vi "Draw Image Frame around marker.vi"(5 "Marker Index":i32, 7 "Camera Settings":T1, 9 "Altitude (m)":dbl, 11 "error in (no error)":errorcluster) -> (15 "error out":errorcluster)   [LabVIEW 2014]
uses:
  C:/Robotic Systems/Products/AgFalcon/Software/Ground Station/Data/Mapping DLL/GMap.NET.WindowsForms.dll
  Data/Mapping DLL/GMap.NET.WindowsForms.dll
  Lat Long Conversion/Controls/PointLatLon.ctl
  C:/Robotic Systems/Products/AgFalcon/Software/Ground Station/Data/Mapping DLL/GMap.NET.Core.dll
  Data/Mapping DLL/GMap.NET.Core.dll
  Reference/SubVI/Main Map Control Refernce.vi
  Settings File/Controls/Camera Settings.ctl
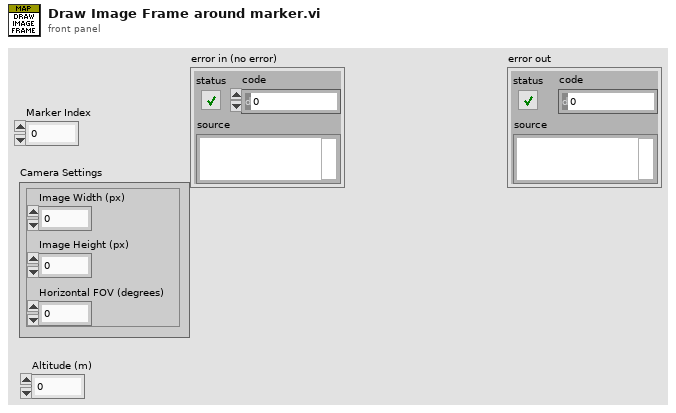
[diagram p1: front panel]
types:
  T1 = typedef "Camera Settings.ctl" = cluster{"Image Width (px)":dbl, "Image Height (px)":dbl, "Horizontal FOV (degrees)":dbl}
  T2 = typedef "PointLatLon.ctl" = cluster{"Longitude":dbl, "Latitude":dbl}
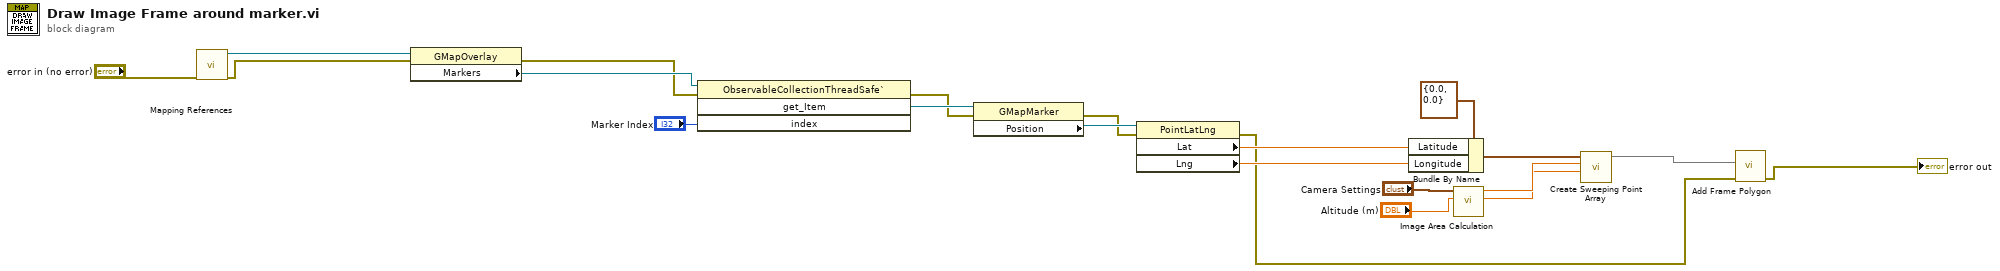
[diagram p0: block diagram]
diagram:
  n1 = call-poly "Mapping References.vi"("Error In"="error in (no error)") -> ("Error Out"=w3:errorcluster, "Main Map Reference"=w2:refnum<k24>)  [unwired: 9 in]
  n2 = property class="GMapOverlay"(reference=w2, error in=w3) -> (error out=w19:errorcluster, "Markers"=w21:refnum<k24>)  [unwired: 1 out]
  n3 = invoke class="ObservableCollectionThreadSafe`" method="get_Item"(reference=w21, error in=w19, "index"="Marker Index") -> (error out=w17:errorcluster, "get_Item"=w18:refnum<k24>)  [unwired: 1 in, 2 out]
  n4 = property class="GMapMarker"(reference=w18, error in=w17) -> (error out=w15:errorcluster, "Position"=w16:refnum<k24>)  [unwired: 1 out]
  n5 = property class="PointLatLng"(reference=w16, error in=w15) -> (error out=w9:errorcluster, "Lat"=w11:dbl, "Lng"=w10:dbl)  [unwired: 1 out]
  n6 = Bundle By Name(cluster=T2 {"Longitude"=0.0, "Latitude"=0.0} ("Origin Point"), "Latitude"=w11, "Longitude"=w10) -> (w7:T2)
  n7 = call "Image Area Calculation.vi"("Altitude (m)"="Altitude (m)", "Camera Settings"="Camera Settings") -> ("Height (m)"=w5:dbl, "Width (m)"=w6:dbl)  [unwired: 6 in, 2 out]
  n8 = call "Create Sweeping Point Array.vi"(9:w5, 10:w6, "Origin Point"=w7) -> (3:w4)  [unwired: 7 in, 1 out]
  n9 = call "Add Frame Polygon.vi"("error in (no error)"=w9, "Point Array"=w4) -> ("error out"=→"error out":errorcluster)  [unwired: 9 in]
